vi "example.vi"() -> ()   [LabVIEW 2025, in "controller.lvclass"]
uses:
  controller.lvclass
  controller.lvclass/controller.ctl
panel:
  in  "dt [s]":dbl
  out "input":dbl
  out "State":dbl
  out "error out":errorcluster
  out "controller out":refnum<class "controller.lvclass">
  in  "Frequncey [Hz]":u16(slide)=1 scale=0.0..10.0
  in  "Reference":dbl(slide) scale=0.0..500.0
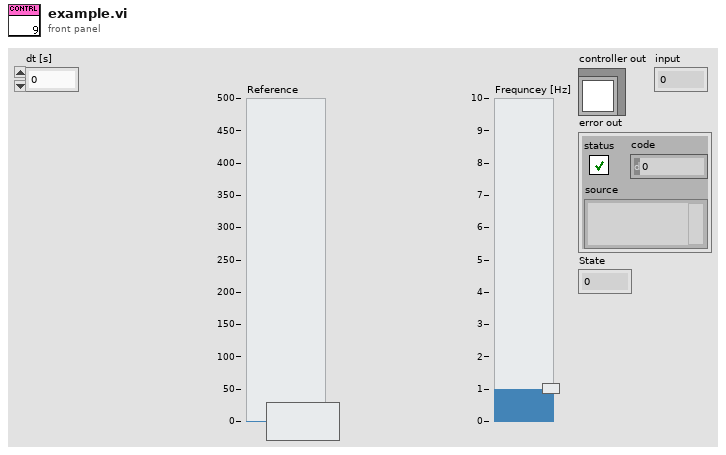
[diagram p1: front panel]
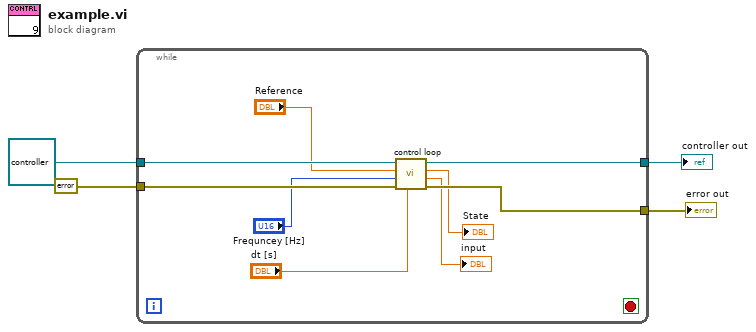
[diagram p0: block diagram]
diagram:
  n1 = while {
    tunnel: refnum<class "controller.lvclass"> refnum ("controller.lvclass") -> [w13]
    tunnel: errorcluster {"status"=FALSE, "code"=0, "source"=""} ("error in (no error)") -> [w12]
    tunnel: [w11] -> w2
    tunnel: [w10] -> w1
    stop <- _ stop-if-true
    n2 = call-dynamic "control loop.vi"("dt [s]"="dt [s]", "error in (no error)"=w12, "Frequncey [Hz]"="Frequncey [Hz]", "Reference"="Reference", "controller in"=w13) -> ("error out"=w10:errorcluster, "input"=→"input":dbl, "State"=→"State":dbl, "controller out"=w11:refnum<class "controller.lvclass">)  [unwired: 3 in]
  }
  "controller out" <- w2
  "error out" <- w1
